vi "Global Loop Reactive.vi"() -> ()   [LabVIEW 2012]
uses:
  <vilib>/Platform/TimedLoop/XDataNode/timing_clust.ctl
  <vilib>/Platform/TimedLoop/XDataNode/nitl_modes.ctl
  <vilib>/Platform/TimedLoop/XDataNode/wakeup.ctl
  Utilities/Robot Parameters/Robot Parameters.vi
  <vilib>/Platform/TimedLoop/XDataNode/XDataNode.xnode
  <vilib>/Platform/TimedLoop/XDataNode/XDNodeRunTimeDep.lvlib
panel:
  in  "stop?":bool
  out "Error Out":errorcluster
  in  "Error In":errorcluster
  out "GPS Waypoint CSV Path":path
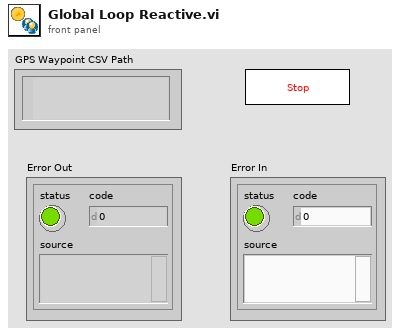
[diagram p1: front panel]
types:
  T1 = cluster{"Latitude":dbl, "Longitude":dbl, "Altitude":dbl, "Velocity, Correction & SET":cluster{"Velocity North":dbl, "Velocity East":dbl, "Velocity Up":dbl, "Ellipsoidal Height":dbl, "GDOP":sgl, "PDOP":sgl, "HDOP":sgl, "VDOP":sgl, "TDOP":sgl, "Horizontal Figure of Merit":u8, "Time Figure of Merit":u8, "Max dGPS Age":sgl, "Extended Navigation Mode":u8, "Antenna Height Adjustment ":dbl, "SET North":i32, "SET East":i32, "SET Up":i32}, "Time":cluster{"GPS Week":u16, "GPS Time of Week":sgl}, "Satellites Used":i32[]}[]
  T2 = cluster{"Latitude":dbl, "Longitude":dbl, "Altitude":dbl, "Velocity, Correction & SET":cluster{"Velocity North":dbl, "Velocity East":dbl, "Velocity Up":dbl, "Ellipsoidal Height":dbl, "GDOP":sgl, "PDOP":sgl, "HDOP":sgl, "VDOP":sgl, "TDOP":sgl, "Horizontal Figure of Merit":u8, "Time Figure of Merit":u8, "Max dGPS Age":sgl, "Extended Navigation Mode":u8, "Antenna Height Adjustment ":dbl, "SET North":i32, "SET East":i32, "SET Up":i32}, "Time":cluster{"GPS Week":u16, "GPS Time of Week":sgl}, "Satellites Used":i32[]}
  T3 = typedef "XDNodeRunTimeDep.lvlib/timing_clust.ctl" = cluster{"Expected End [f-1]":u64, "Actual End [f-1]":u64, "Finished Late? [f-1]":bool, "Expected End [i-1]":u64, "Actual End [i-1]":u64, "Finished Late? [i-1]":bool, "Expected Start [i]":u64, "Actual Start [i]":u64, "Expected Start [f]":u64, "Actual Start [f]":u64, "Source Name":string, "Structure Name":string, "Period":i64, "Deadline":i64, "Offset":i64, "Start":i64, "Priority":i32, "Timeout":i32, "Mode":T4, "Wakeup Reason":T5, "Error":errorcluster, "Source Type":string, "Secondary Source Type":string, "Global End Time":u64, "Global Start Time":u64, "Frame Duration":u64, "Iteration Duration":u64, "Assigned CPU":i32, "I/O Scan Engine Mode":u32}
  T4 = typedef "XDNodeRunTimeDep.lvlib/nitl_modes.ctl" = enum32{"No Change", "Process missed periods, maintain original phase", "Discard missed periods, maintain original phase", "Process missed periods, ignore original phase", "Discard missed periods, ignore original phase"}
  T5 = typedef "XDNodeRunTimeDep.lvlib/wakeup.ctl" = enum32{"Normal", "Aborted", "Asynchronous wakeup", "Timing source error", "Timed loop error", "Timeout"}
  T6 = enum16{"Idle", "Wiimote", "Joypad", "IGVC", "Avoide Objects", "Avoide Lines", "Path Planning", "Heading", "Waypoint"}
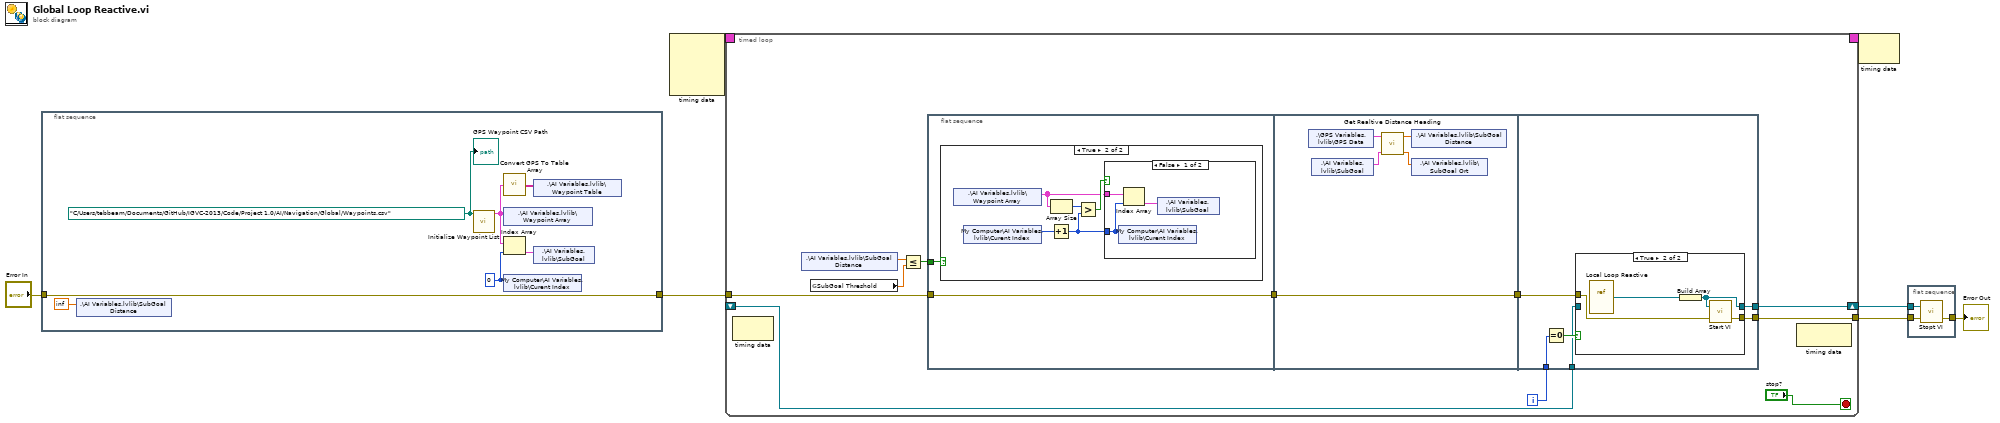
[diagram p0: block diagram]
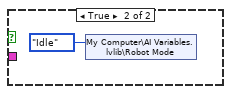
[diagram p3: hidden frame]
diagram:
  n1 = flat-sequence {
    tunnel: "Error In" -> [w14]
    tunnel: [w14] -> w4
    frame #0 {
      w8 = path "C:/Users/tebbeam/Documents/GitHub/IGVC-2013/Code/Project 1.0/AI/Navigation/Global/Waypoints.csv" ("GPS Waypoint CSV Path")
      w9 = 0 ("index")
      n2 = shared-variable ".\\AI Variables.lvlib\\SubGoal Distance"(inf) -> ()  [unwired: 1 in, 1 out]
      n3 = call "Initialize Waypoint List.vi"("GPS Waypoint CSV Path"=w8) -> ("Waypoint Array"=w13:T1)  [unwired: 10 in]
      n4 = call "Convert GPS To Table Array.vi"("Waypoint Array In"=w13) -> ("Lat/Long Array Out"=w12:string[][])
      n5 = shared-variable ".\\AI Variables.lvlib\\Waypoint Array"(w13) -> ()  [unwired: 1 in, 1 out]
      n6 = Index Array(array=w13, index=w9) -> (element=w10:T2)
      n7 = shared-variable "My Computer\\AI Variables.lvlib\\Curent Index"(w9) -> ()  [unwired: 1 in, 1 out]
      n8 = shared-variable ".\\AI Variables.lvlib\\Waypoint Table"(w12) -> ()  [unwired: 1 in, 1 out]
      n9 = shared-variable ".\\AI Variables.lvlib\\SubGoal"(w10) -> ()  [unwired: 1 in, 1 out]
      "GPS Waypoint CSV Path" <- w8
    }
  }
  n10 = node-c288() -> (w6:T3)  [unwired: 4 in]
  n11 = timed-loop {
    timing: w6 -> [_]
    timing-out: [_] -> w5
    tunnel: w4 -> [w22]
    tunnel: [w21] -> w3
    shift-right: [w23] -> w1
    shift-left: _ -> [w20]
    i -> [w24]
    stop <- "stop?" stop-if-true
    n12 = node-c288() -> ()  [unwired: 1 in, 1 out]
    n13 = shared-variable ".\\AI Variables.lvlib\\SubGoal Distance"() -> (w19:dbl)  [unwired: 1 in, 1 out]
    n14 = global read "Robot Parameters.vi" "SubGoal Threshold"() -> (w18:dbl)
    n15 = Less Or Equal?(x=w19, y=w18) -> (x <= y?=w17:bool)
    n16 = flat-sequence {
      tunnel: w22 -> [w27]
      tunnel: [w27] -> w16
      tunnel: w17 -> [w26]
      tunnel: w16 -> [w41]
      tunnel: [w41] -> w15
      tunnel: w24 -> [w46]
      tunnel: [w45] -> w23
      tunnel: [w43] -> w21
      tunnel: w20 -> [w42]
      tunnel: w15 -> [w44]
      frame #0 {
        n17 = case shown="True" w26 {
          frame False {
          }
          frame True {
            n18 = shared-variable ".\\AI Variables.lvlib\\Waypoint Array"() -> (w28:T1)  [unwired: 1 in, 1 out]
            n19 = shared-variable "My Computer\\AI Variables.lvlib\\Curent Index"() -> (w32:i32)  [unwired: 1 in, 1 out]
            n20 = Array Size(array=w28) -> (size(s)=w31:i32)
            n21 = Increment(x=w32) -> (x+1=w29:i32)
            n22 = Greater?(x=w31, y=w29) -> (0:w30:bool)
            n23 = case shown="False" w30 {
              tunnel: w28 -> [w34 _]
              tunnel: w29 -> [w33 _]
              frame False {
                n24 = shared-variable "My Computer\\AI Variables.lvlib\\Curent Index"(w33) -> ()  [unwired: 1 in, 1 out]
                n25 = Index Array(array=w34, index=w33) -> (element=w35:T2)
                n26 = shared-variable ".\\AI Variables.lvlib\\SubGoal"(w35) -> ()  [unwired: 1 in, 1 out]
              }
              frame True {
                n27 = shared-variable "My Computer\\AI Variables.lvlib\\Robot Mode"(T6."Idle" ("Robot Mode")) -> ()  [unwired: 1 in, 1 out]
              }
            }
          }
        }
      }
      frame #1 {
        n28 = shared-variable ".\\GPS Variables.lvlib\\GPS Data"() -> (w37:T2)  [unwired: 1 in, 1 out]
        n29 = shared-variable ".\\AI Variables.lvlib\\SubGoal"() -> (w38:T2)  [unwired: 1 in, 1 out]
        n30 = call "Get Realtive Distance Heading.vi"("Goal Position"=w38, "Current Position"=w37) -> ("Bearing"=w40:dbl, "distance (m)"=w39:dbl)  [unwired: 8 in]
        n31 = shared-variable ".\\AI Variables.lvlib\\SubGoal Distance"(w39) -> ()  [unwired: 1 in, 1 out]
        n32 = shared-variable ".\\AI Variables.lvlib\\SubGoal Ort"(w40) -> ()  [unwired: 1 in, 1 out]
      }
      frame #2 {
        n33 = Equal To 0?(x=w46) -> (x = 0?=w47:bool)
        n34 = case shown="True" w47 {
          tunnel: [w49 w52] -> w43
          tunnel: [w48 w51] -> w45
          tunnel: w44 -> [w49 w50]
          tunnel: w42 -> [w48 _]
          frame False {
          }
          frame True {
            n35 = vi-ref "Local Loop Reactive.vi"() -> (w53:refnum<vi>)
            n36 = Build Array(w53) -> (w51:refnum<vi>[])
            n37 = call "Start VI.vi"("error in"=w50, "VI refnum"=w51) -> ("error out"=w52:errorcluster)  [unwired: 1 in]
          }
        }
      }
    }
    n38 = node-c288() -> ()  [unwired: 1 in, 1 out]
  }
  n39 = node-c288(w5) -> ()  [unwired: 1 out]
  n40 = flat-sequence {
    tunnel: w3 -> [w58]
    tunnel: [w57] -> w2
    tunnel: w1 -> [w56]
    frame #0 {
      n41 = call "Stopt VI.vi"("error in"=w58, "VI refnum"=w56) -> ("error out"=w57:errorcluster)  [unwired: 1 in]
    }
  }
  "Error Out" <- w2
